vi "CreateRotatedAndFlippedImage.vi"(8 "Error In":errorcluster, 11 "ImageIn":T1={"Id"=0, "Image"=[[FALSE, TRUE, FALSE, FALSE, FALSE, FALSE, FALSE, FALSE, FALSE, TRUE], [TRUE, TRUE, FALSE, FALSE, FALSE, FALSE, FALSE, FALSE, FALSE, FALSE], [FALSE, FALSE, FALSE, FALSE, FALSE, FALSE, FALSE, FALSE, FALSE, FALSE], [FALSE, FALSE, FALSE, FALSE, FALSE, FALSE, FALSE, FALSE, FALSE, FALSE], [FALSE, FALSE, FALSE, FALSE, FALSE, FALSE, FALSE, FALSE, FALSE, FALSE], [FALSE, FALSE, FALSE, FALSE, FALSE, FALSE, FALSE, FALSE, FALSE, FALSE], [TRUE, TRUE, TRUE, TRUE, FALSE, FALSE, FALSE, FALSE, FALSE, FALSE], [FALSE, FALSE, FALSE, TRUE, FALSE, FALSE, FALSE, TRUE, TRUE, TRUE], [FALSE, FALSE, FALSE, TRUE, FALSE, FALSE, FALSE, TRUE, FALSE, FALSE], [FALSE, FALSE, FALSE, TRUE, FALSE, FALSE, FALSE, TRUE, FALSE, FALSE]]}) -> (0 "Error Out":errorcluster, 3 "RotatedAndFlipped":T1[](array[typedef]))   [LabVIEW 2020, in "2020_20.lvclass"]
uses:
  2020_20.lvclass
  Image.ctl
panel:
  out "Flipped(Hor)":T1[](array[typedef])
  out "Rotated":T1[](array[typedef])
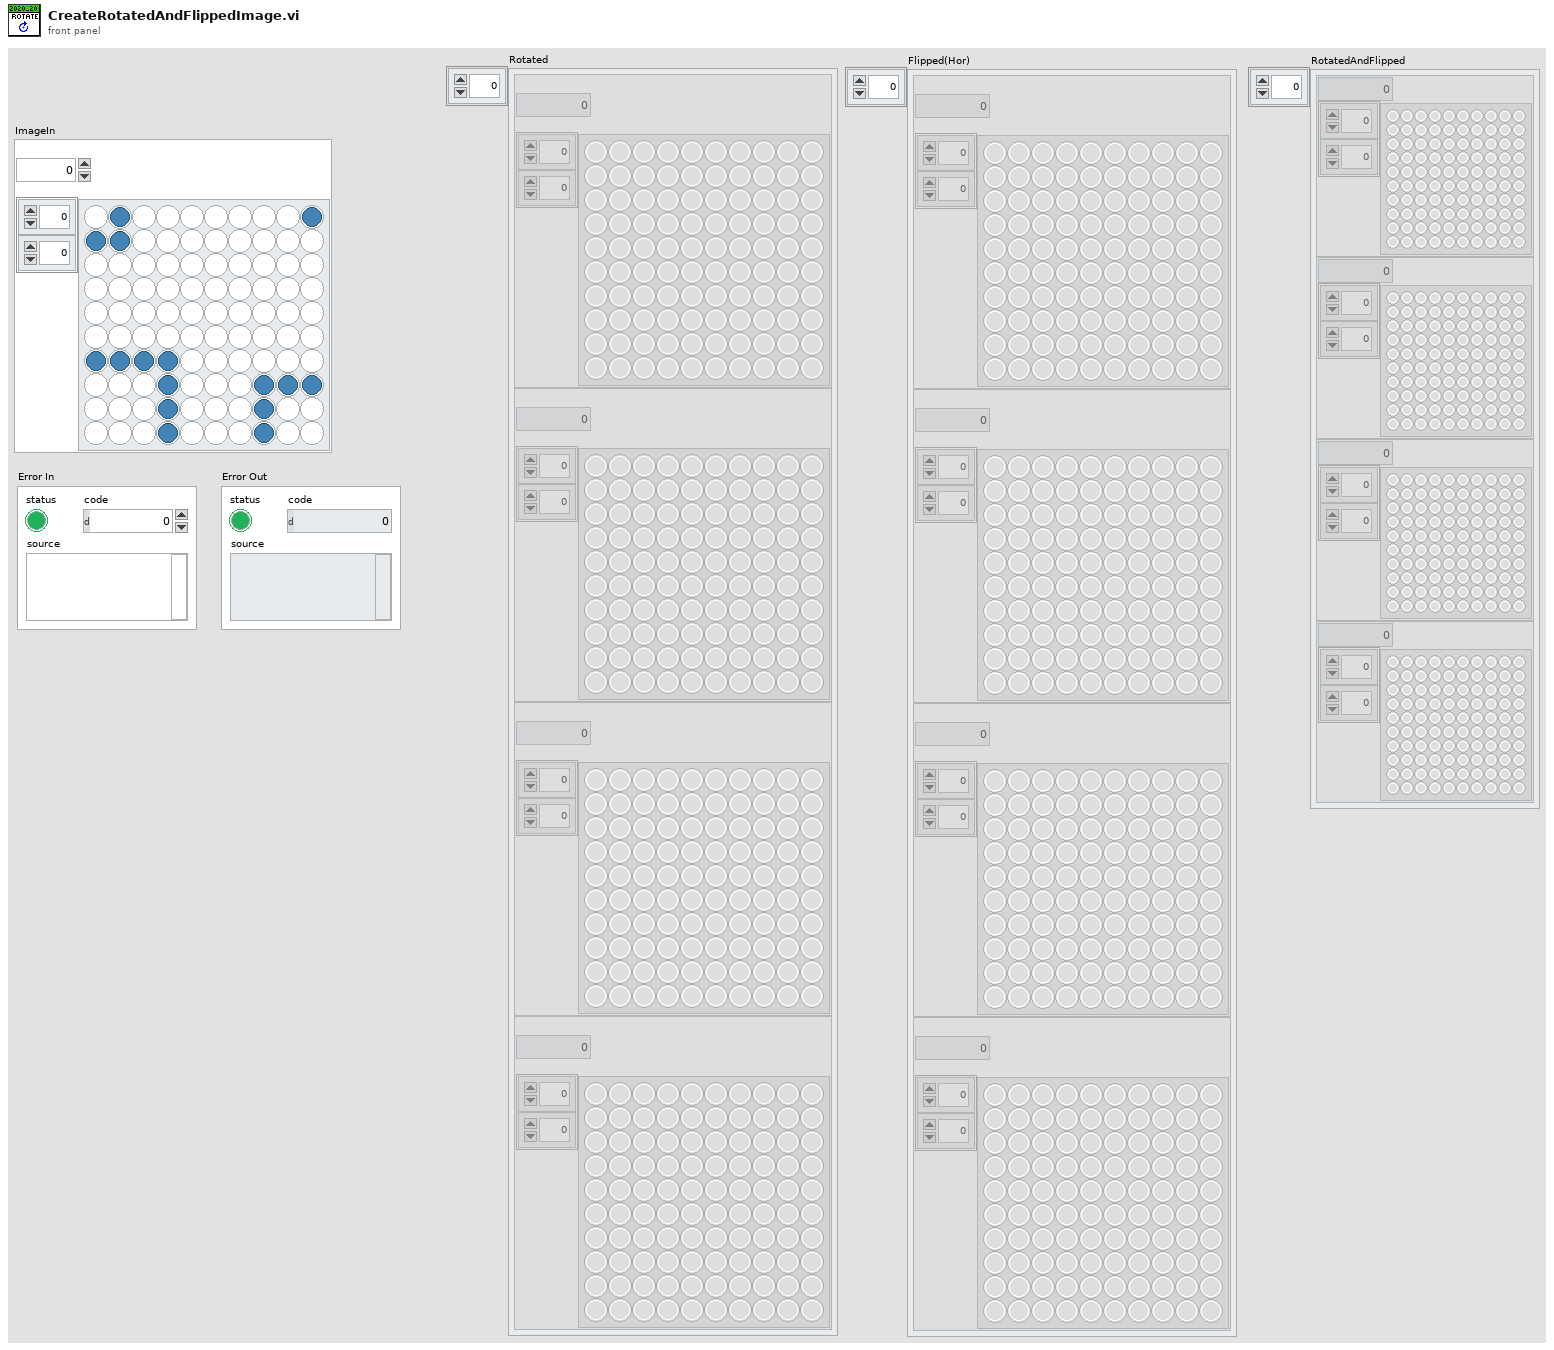
[diagram p1: front panel]
types:
  T1 = typedef "2020_20.lvclass/Image.ctl" = cluster{"Id":i32, "Image":bool[][]}
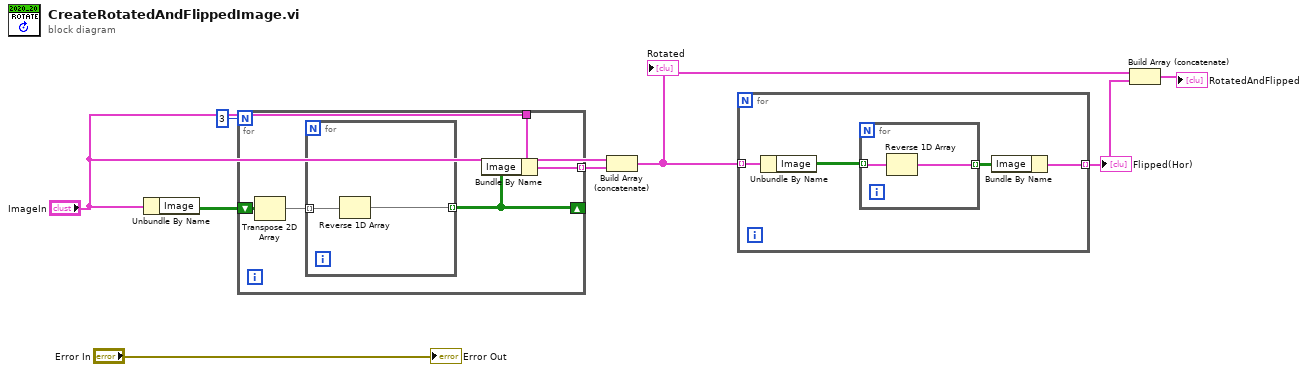
[diagram p0: block diagram]
diagram:
  n1 = Unbundle By Name("ImageIn") -> ("Image"=w7:bool[][])
  n2 = for {
    N: 3 -> [_]
    tunnel: "ImageIn" -> [w13]
    shift-right: [w10] -> _
    shift-left: w7 -> [w12]
    tunnel: [w9] -> w5 mode=indexing
    n3 = Transpose 2D Array(2D array=w12) -> (transposed array=w11:bool[][])
    n4 = for {
      tunnel: w11 -> [w15] mode=indexing
      tunnel: [w14] -> w10 mode=indexing
      n5 = Reverse 1D Array(array=w15) -> (reversed array=w14:bool[])
    }
    n6 = Bundle By Name(cluster=w13, "Image"=w10) -> (w9:T1)
  }
  n7 = Build Array (concatenate)("ImageIn", w5) -> (w3:T1[])
  "Rotated" <- w3
  n8 = for {
    tunnel: w3 -> [w16] mode=indexing
    tunnel: [w18] -> w2 mode=indexing
    n9 = Unbundle By Name(w16) -> ("Image"=w17:bool[][])
    n10 = for {
      tunnel: w17 -> [w21] mode=indexing
      tunnel: [w20] -> w19 mode=indexing
      n11 = Reverse 1D Array(array=w21) -> (reversed array=w20:bool[])
    }
    n12 = Bundle By Name(cluster=w16, "Image"=w19) -> (w18:T1)
  }
  "Flipped(Hor)" <- w2
  n13 = Build Array (concatenate)(w3, w2) -> (→"RotatedAndFlipped":T1[])
  "Error Out" <- "Error In"
